vi "Main.vi"(5 "Deliminated Char":string=".", 6 "Folder names":string[](array[string])=["StaARx#[PLC]StaATesterRxSignals", "StaATx#[PLC]StaATesterTxSignals"], 7 "PLC FGVname":string="OPC Ref", 8 "error in":errorcluster, 9 "Sequence Context In":refnum<k7>, 10 "Event Sources":T1, 11 "PreUUT In":refnum<class "PreUUT.lvclass">) -> (0 "error out":errorcluster, 2 "Station":string="asdfasdf", 3 "OPC UA Out":refnum<class "PreUUT.lvclass">)   [LabVIEW 2021, in "PreUUT.lvclass"]
uses:
  PreUUT.lvclass
  Controls/Rx PreUUT.ctl
  Controls/Tx PreUUT.ctl
  PreUUT.lvclass/PreUUT.ctl
  <vilib>/addons/TestStand/_TSUtility.llb/TestStand - Get Property Value (Number {Signed 32-bit Integer}).vi
  OPC UA/OPC UA.lvclass
panel:
  out "Connect?":bool
  in  "Tx PreUUT":T2={"Online"=TRUE, "Ready"=TRUE, "Fault"=FALSE, "Timeout"=FALSE, "Results"=0, "StepNo"=0, "TestRunning"=FALSE, "ResultsReady"=FALSE}
  out "Rx PreUUT":T3
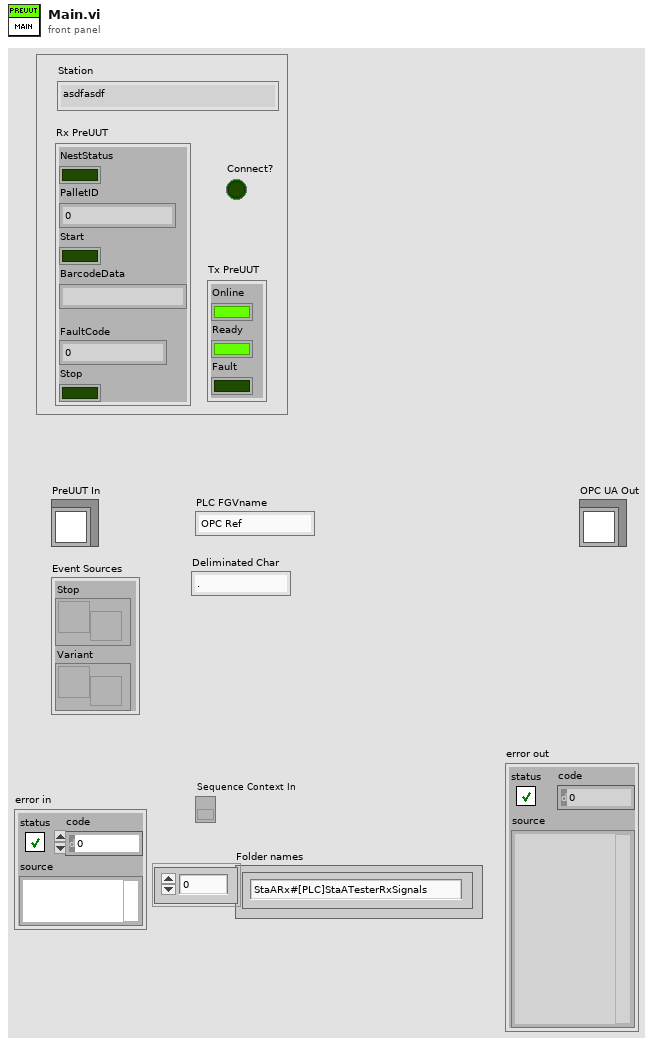
[diagram p1: front panel]
types:
  T1 = cluster{"Stop":refnum<user-event>, "Variant":refnum<user-event>}
  T2 = typedef "PreUUT.lvclass/Tx PreUUT.ctl" = cluster{"Online":bool, "Ready":bool, "Fault":bool, "Timeout":bool, "Results":u32, "StepNo":u32, "TestRunning":bool, "ResultsReady":bool}
  T3 = typedef "PreUUT.lvclass/Rx PreUUT.ctl" = cluster{"NestStatus":bool, "PalletID":u32, "Start":bool, "BarcodeData":string, "FaultCode":u32, "Stop":bool}
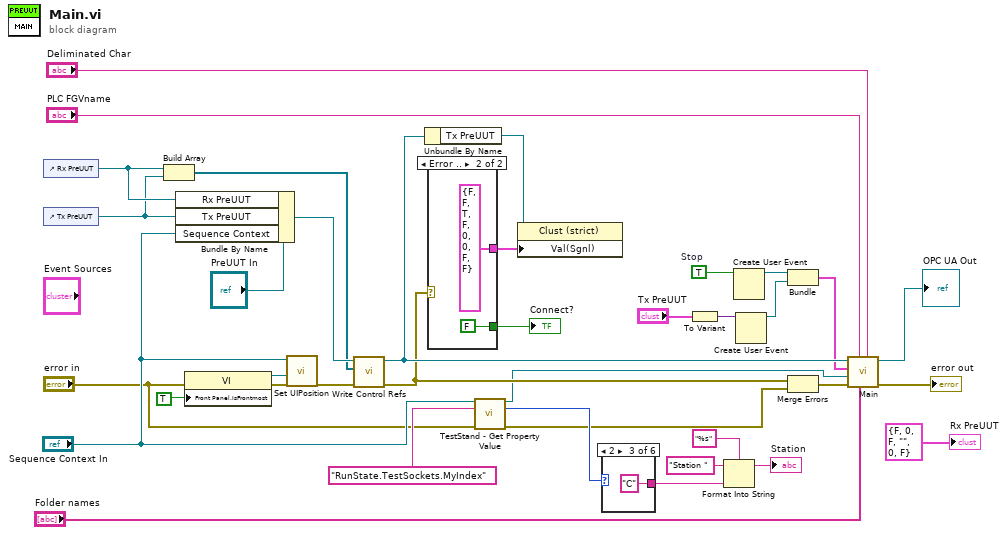
[diagram p0: block diagram]
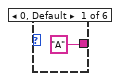
[diagram p2: hidden frame]
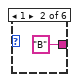
[diagram p3: hidden frame]
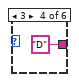
[diagram p4: hidden frame]
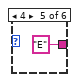
[diagram p5: hidden frame]
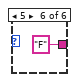
[diagram p6: hidden frame]
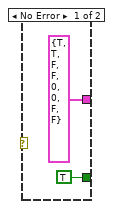
[diagram p7: hidden frame]
diagram:
  w25 = TRUE  # Stop
  n1 = control-ref of="Rx PreUUT"() -> (w32:refnum<vi>)
  n2 = control-ref of="Tx PreUUT"() -> (w31:refnum<vi>)
  n3 = Build Array(w32, w31) -> (w30:refnum<vi>[])
  n4 = Bundle By Name(cluster="PreUUT In", "Rx PreUUT"=w32, "Tx PreUUT"=w31, "Sequence Context"="Sequence Context In") -> (w33:refnum<class "PreUUT.lvclass">)
  n5 = property class="VI"(error in="error in", "Front Panel.IsFrontmost"=TRUE ("Front Panel Window:Is Frontmost")) -> (reference out=w17:refnum<vi>, error out=w18:errorcluster)  [unwired: 1 in]
  n6 = call "Set UIPosition.vi"("error in"=w18, "VI Ref"=w17, "Sequence Context In"="Sequence Context In") -> ("error out"=w19:errorcluster)  [unwired: 8 in]
  n7 = call-dynamic "Write Control Refs.vi"("error in (no error)"=w19, "Ctl Refs"=w30, "OPC UA in"=w33) -> ("error out"=w2:errorcluster, "OPC UA out"=w22:refnum<class "PreUUT.lvclass">)  [unwired: 7 in]
  n8 = Unbundle By Name(w22) -> ("Tx PreUUT"=w35:refnum<vi>)
  n9 = case shown="Error .." w2 {
    tunnel: [T2 {"Online"=TRUE, "Ready"=TRUE, "Fault"=FALSE, "Timeout"=FALSE, "Results"=0, "StepNo"=0, "TestRunning"=FALSE, "ResultsReady"=FALSE} ("Tx PreUUT") T2 {"Online"=FALSE, "Ready"=FALSE, "Fault"=TRUE, "Timeout"=FALSE, "Results"=0, "StepNo"=0, "TestRunning"=FALSE, "ResultsReady"=FALSE} ("Tx PreUUT")] -> w36
    tunnel: [TRUE ("Connect?") FALSE ("Connect?")] -> w20
    frame No Error {
    }
    frame Error {
    }
  }
  "Connect?" <- w20
  n10 = call-poly <vilib>:"TestStand - Get Property Value.vi"("Sequence Context In"="Sequence Context In", "Lookup String"="RunState.TestSockets.MyIndex", "error in (no error)"="error in") -> ("Sequence Context Out"=w1:refnum<k7>, "Value"=w11:i32, "error out"=w6:errorcluster)  [unwired: 10 in]
  n11 = property class="Clust (strict)"(reference=w35, "Val(Sgnl)"=w36) -> ()  [unwired: 1 in, 2 out]
  n12 = case shown="2" w11 {
    tunnel: ["A" ("format string") "B" ("format string") "C" ("format string") "D" ("format string") "E" ("format string") "F" ("format string")] -> w12
    frame 0, Default {
    }
    frame 1 {
    }
    frame 2 {
    }
    frame 3 {
    }
    frame 4 {
    }
    frame 5 {
    }
  }
  n13 = To Variant(anything="Tx PreUUT") -> (Variant=w27:variant)
  n14 = Format Into String(format string="%s", initial string="Station ", w12) -> (resulting string=→"Station":string)  [unwired: 1 in, 1 out]
  n15 = Create User Event(user event datatype=w25) -> (user event=w24:refnum<user-event>)  [unwired: 1 in, 1 out]
  n16 = Create User Event(user event datatype=w27) -> (user event=w26:refnum<user-event>)  [unwired: 1 in, 1 out]
  n17 = Bundle("Stop"=w24, "Variant"=w26) -> (w15:T1)  [unwired: 1 in]
  n18 = Merge Errors(w2, w6) -> (w3:errorcluster)
  n19 = call-parent "Main.vi"("Deliminated Char"="Deliminated Char", "Folder names"="Folder names", "FGVname"="PLC FGVname", "error in"=w3, "Sequence Context In"=w1, "Event Sources"=w15, "OPC UA In"=w22) -> ("error out"=→"error out":errorcluster, "OPC UA Out"=→"OPC UA Out":refnum<class "PreUUT.lvclass">)  [unwired: 2 in, 1 out]
  "Rx PreUUT" <- T3 {"NestStatus"=FALSE, "PalletID"=0, "Start"=FALSE, "BarcodeData"="", "FaultCode"=0, "Stop"=FALSE} ("Rx PreUUT")
